vi "Set Element At (Dimensions).vi"(8 "error in (no error)":errorcluster, 9 "Element":refnum<class "Data.lvclass">, 10 "Index":i32[](array[numeric]), 11 "Array in":refnum<class "Array.lvclass">) -> (0 "error out":errorcluster, 3 "Array out":refnum<class "Array.lvclass">)   [LabVIEW 2012, in "MDSplus.lvlib" / "Array.lvclass"]
uses:
  <vilib>/MDSplus/Classes/Data_Class/Array_Class/Array.lvclass
  <vilib>/MDSplus/Classes/Data_Class/Data.lvclass
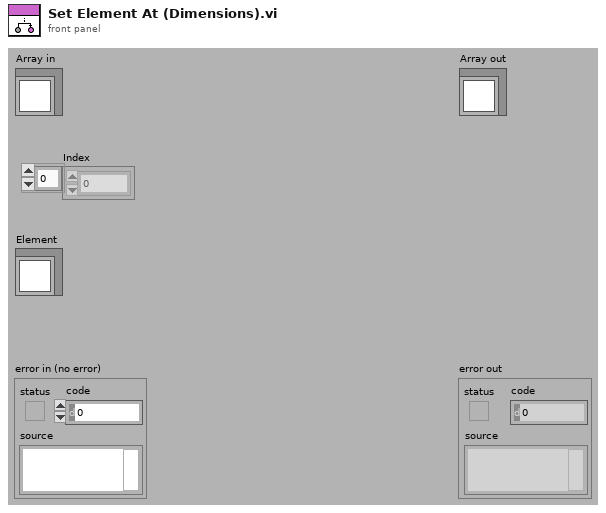
[diagram p1: front panel]
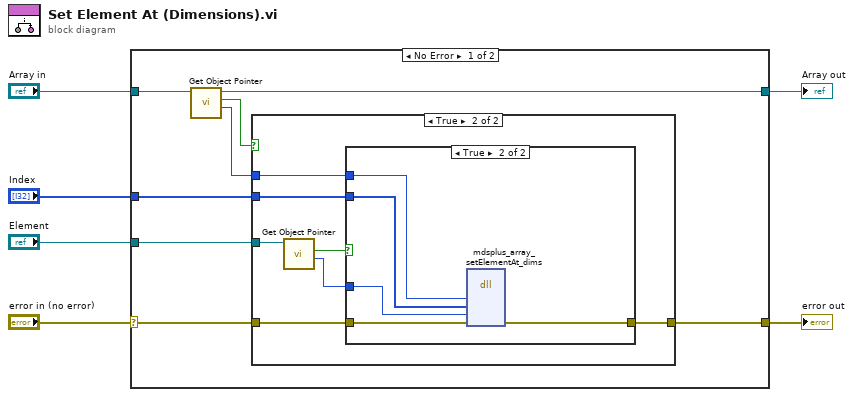
[diagram p0: block diagram]
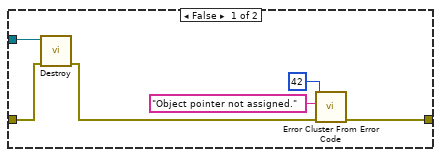
[diagram p2: hidden frame]
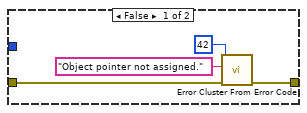
[diagram p3: hidden frame]
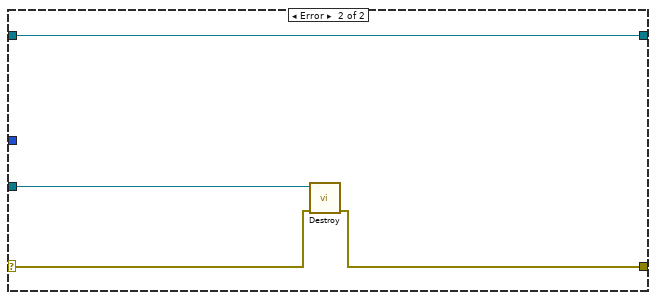
[diagram p4: hidden frame]
diagram:
  n1 = case shown="No Error" "error in (no error)" {
    selector: "error in (no error)" -> [w9 w38]
    tunnel: [w8 w37] -> w5
    tunnel: [w7 w40] -> w3
    tunnel: "Array in" -> [w14 w40]
    tunnel: "Index" -> [w13 _]
    tunnel: "Element" -> [w12 w39]
    frame No Error {
      n2 = call-dynamic "Get Object Pointer.vi"("Data in"=w14) -> ("Object Pointer"=w10:i64, "Assigned object pointer?"=w11:bool, "Data out"=w7:refnum<class "Array.lvclass">)  [unwired: 8 in]
      n3 = case shown="True" w11 {
        tunnel: w13 -> [_ w27]
        tunnel: w12 -> [w17 w26]
        tunnel: w10 -> [_ w23]
        tunnel: w9 -> [w16 w22]
        tunnel: [w18 w21] -> w8
        frame False {
          n4 = call-dynamic "Destroy.vi"("error in (no error)"=w16, "Data in"=w17) -> ("error out"=w15:errorcluster)  [unwired: 9 in]
          n5 = call <vilib>:"Error Cluster From Error Code.vi"("error in (no error)"=w15, "error message (\"\")"="Object pointer not assigned." ("error message (\"\")"), "error code (0)"=42) -> ("error out"=w18:errorcluster)  [unwired: 6 in]
        }
        frame True {
          n6 = call-dynamic "Get Object Pointer.vi"("Data in"=w26) -> ("Object Pointer"=w24:i64, "Assigned object pointer?"=w25:bool)  [unwired: 8 in, 1 out]
          n7 = case shown="True" w25 {
            tunnel: w27 -> [_ w35]
            tunnel: w24 -> [_ w34]
            tunnel: w23 -> [_ w36]
            tunnel: w22 -> [w29 w33]
            tunnel: [w28 w32] -> w21
            frame False {
              n8 = call <vilib>:"Error Cluster From Error Code.vi"("error in (no error)"=w29, "error message (\"\")"="Object pointer not assigned." ("error message (\"\")"), "error code (0)"=42) -> ("error out"=w28:errorcluster)  [unwired: 6 in]
            }
            frame True {
              n9 = dll-call lib="MDSobjectsLVShr" fn="mdsplus_array_setElementAt_dims"("lvArrayPtr"=w36, "lvIntArrHdlIn"=w35, "lvDataPtrIn"=w34, "error"=w33) -> ("error"=w32:errorcluster)  [unwired: 7 in, 2 out]
            }
          }
        }
      }
    }
    frame Error {
      n10 = call-dynamic "Destroy.vi"("error in (no error)"=w38, "Data in"=w39) -> ("error out"=w37:errorcluster)  [unwired: 9 in]
    }
  }
  "error out" <- w5
  "Array out" <- w3
